vi "ELOG_Calculations_Set.vi"(8 "error in (no error)":errorcluster, 10 "Calculation Mode":string[](array[combo]), 11 "OXY_SCPI Reseource In":refnum<visa-resource-name>) -> (0 "error out":errorcluster, 1 "communication_data":T1, 3 "OXY_SCPI Reseource Out":refnum<visa-resource-name>)   [LabVIEW 2018, in "OXYGEN.lvlib"]
doc: "Sets a list of requested statistical calculations for all channels"
uses:
  OXYGEN.lvlib
  TypeDefs/Cluster_RawCommData.ctl
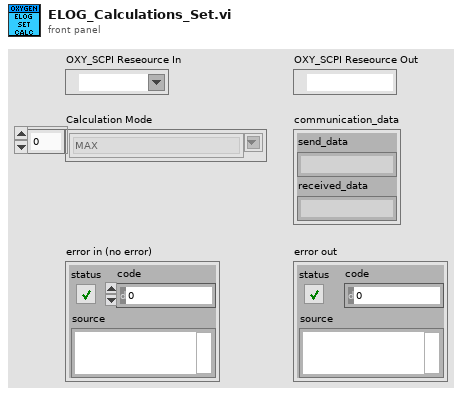
[diagram p1: front panel]
types:
  T1 = typedef "OXYGEN.lvlib/Cluster_RawCommData.ctl" = cluster{"send_data":string, "received_data":string}
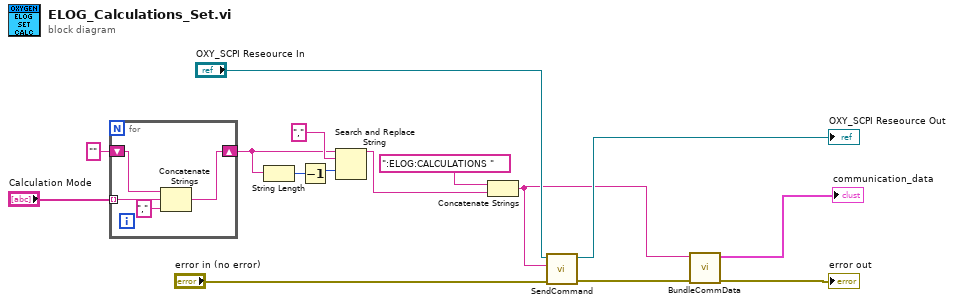
[diagram p0: block diagram]
diagram:
  n1 = for {
    tunnel: "Calculation Mode" -> [w19] mode=indexing
    shift-right: [w17] -> w4
    shift-left: "" -> [w16]
    n2 = Concatenate Strings(w16, w19, "," ("string")) -> (w17:string)
  }
  n3 = String Length(string=w4) -> (length=w5:i32)
  n4 = Decrement(x=w5) -> (x-1=w7:i32)
  n5 = Search and Replace String(input string=w4, search string=",", offset=w7) -> (result string=w1:string)  [unwired: 5 in, 3 out]
  n6 = Concatenate Strings(":ELOG:CALCULATIONS " ("string"), w1) -> (w12:string)
  n7 = call "SendCommand.vi"("error in (no error)"="error in (no error)", "String to Send"=w12, "OXY_SCPI Reseource In"="OXY_SCPI Reseource In") -> ("error out"=w9:errorcluster, "OXY_SCPI Reseource Out"=→"OXY_SCPI Reseource Out":refnum<visa-resource-name>)  [unwired: 7 in]
  n8 = call "BundleCommData.vi"("error in (no error)"=w9, "send_data"=w12) -> ("error out"=→"error out":errorcluster, "communication_data"=→"communication_data":T1)  [unwired: 8 in]
